vi "Write Data Arr Refnum.vi"(8 "error in (no error)":errorcluster, 10 "Data Arr Refnum":refnum<vi>, 11 "WT1600 in":refnum<class "WT1600.lvclass">) -> (0 "error out":errorcluster, 3 "WT1600 out":refnum<class "WT1600.lvclass">)   [LabVIEW 2013, in "Universal Power Meter.lvlib" / "WT1600.lvlib" / "WT1600.lvclass"]
uses:
  WT1600.lvclass
  WT1600.lvclass/WT1600.ctl
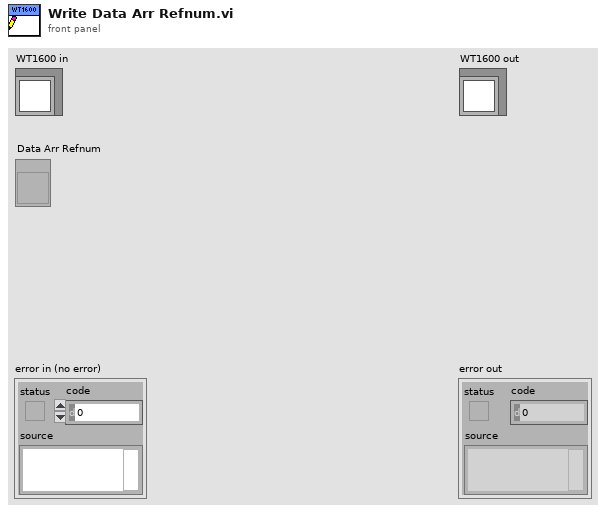
[diagram p1: front panel]
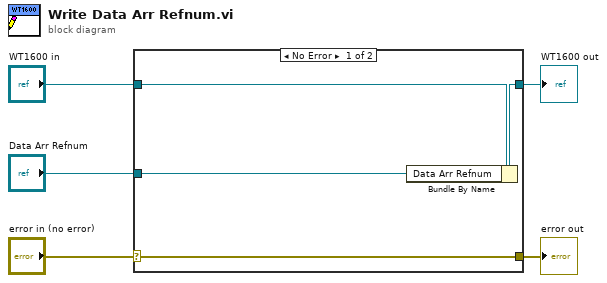
[diagram p0: block diagram]
diagram:
  n1 = case shown="No Error" "error in (no error)" {
    selector: "error in (no error)" -> [w9 w10]
    tunnel: [w9 w10] -> w4
    tunnel: [w7 w11] -> w2
    tunnel: "WT1600 in" -> [w8 w11]
    tunnel: "Data Arr Refnum" -> [w6 _]
    frame No Error {
      n2 = Bundle By Name(cluster=w8, "Data Arr Refnum"=w6) -> (w7:refnum<class "WT1600.lvclass">)
    }
    frame Error {
    }
  }
  "error out" <- w4
  "WT1600 out" <- w2
